vi "Swabian_UI.vi"() -> ()   [LabVIEW 2018]
uses:
  swabian_vis/swabian_channel_settings.ctl
  swabian_vis/channel_settings.ctl
  swabian_vis/reference_checkbox_tdef.ctl
  swabian_vis/stream_modes.ctl
  swabian_vis/swabian_q_tdef.ctl
  swabian_vis/swabian_actions.ctl
  swabian_vis/swabian_local_data_tdef.ctl
  swabian_vis/swabian_events_tdef.ctl
  swabian_vis/update_chart_tdef.ctl
  swabian_vis/channel_data_tdef.ctl
  swabian_vis/swabian_buffer_tdef.ctl
  swabian_vis/leftovers_struct.ctl
  swabian_vis/swabian_hisotgram_settings.ctl
  C:/Users/SWIR TCSPC/Desktop/Swabian/lib/TTCSharp32.dll
  lib/TTCSharp32.dll
panel:
  out "status":string="Status: " caption="Status"
  in  "connect":bool
  in  "experiments":T1(tab)
  in  "Trigger edge":bool[](array[boolean])=[FALSE, FALSE, FALSE, FALSE, FALSE, FALSE, FALSE, FALSE]
  in  "Channels to chart":bool[](array[boolean])=[FALSE, FALSE, FALSE, FALSE, FALSE, FALSE, FALSE, FALSE]
  in  "save_settings":bool
  in  "swabian_channel_settings":T2=[{"Threshold (V)"=0.5, "Input Delay (ps)"=0, "Dead Time (ps)"=6000}, {"Threshold (V)"=0.5, "Input Delay (ps)"=0, "Dead Time (ps)"=6000}, {"Threshold (V)"=0.5, "Input Delay (ps)"=0, "Dead Time (ps)"=6000}, {"Threshold (V)"=0.5, "Input Delay (ps)"=0, "Dead Time (ps)"=6000}, {"Threshold (V)"=0.5, "Input Delay (ps)"=0, "Dead Time (ps)"=6000}, {"Threshold (V)"=0.5, "Input Delay (ps)"=0, "Dead Time (ps)"=6000}, {"Threshold (V)"=0.5, "Input Delay (ps)"=0, "Dead Time (ps)"=6000}, {"Threshold (V)"=0.5, "Input Delay (ps)"=0, "Dead Time (ps)"=6000}] {"Dead Time (ps)" min=0 step=6000; "Threshold (V)" min=0.0 max=2.5 step=0.1}
  in  "chart_counts":bool
  in  "Trigger \nedge":bool[](array[boolean])=[FALSE, FALSE, FALSE, FALSE, FALSE, FALSE, FALSE, FALSE]
  in  "check_sync":bool
  in  "Time (sec)":i64=10 min=1
  in  "Stream Mode":T4
  in  "Notes":string caption="Status"
  in  "Data Path":path=path "C:/Users/SWIR TCSPC/Desktop/Swabian/test_data/test1.photons"
  in  "Channels\nto Stream":bool[](array[boolean])=[TRUE, TRUE, FALSE, FALSE, FALSE, FALSE, FALSE, FALSE]
  in  "stream_to_file":bool
  in  "Reference\nChannel":T5=enum."ch0"
  in  "Sync Rate (Hz)":dbl=40000000.0 min=0.0
  in  "n_bins":i32=100 caption="Number of Bins" min=0
  in  "stop_time":dbl=100.0 caption="Stop time (ns)" min=0.001 max=1000000000.0
  in  "start_time":dbl=1.0 caption="Start Time (ns)" min=0.001 max=1000000000.0
  in  "Time (sec)":i64=1 min=1
  in  "Stream Mode":T4
  in  "Notes":string="Status: " caption="Status"
  in  "Data Path":path=path "C:/Users/bspoka/Desktop/phot_test.photons"
  in  "Channels to\nHistogram":bool[](array[boolean])=[FALSE, FALSE, FALSE, FALSE, FALSE, FALSE, FALSE, FALSE]
  in  "plot_lifetimes":bool
  in  "Reference\nChannel":T5
  in  "sync_rate_histo":i32 caption="Sync Rate (Hz)" min=0
  in  "plots":enum32{"chart", "xy_graph"}(tab)
  out "counts_chart":T6(graph)
  out "Counts/sec":T6
  in  "save_chart_data":bool
  out "xy_graph":cluster{dbl[], dbl[]}[](graph)
  # "0"
  # "1"
  # "2"
  # "3"
  # "4"
  # "5"
  # "6"
  # "7"
  # "Threshold (V)"
  # "Delay (ps)"
  # "Dead Time (ps)"
  # "Ch 0"
  # "Ch 1"
  # "Ch 2"
  # "Ch 3"
  # "Ch 4"
  # "Ch 5"
  # "Ch 6"
  # "Ch 7"
  # "0"
  # "1"
  # "2"
  # "3"
  # "4"
  # "5"
  # "6"
  # "7"
  # "0"
  # "1"
  # "2"
  # "3"
  # "4"
  # "5"
  # "6"
  # "7"
  # "0"
  # "1"
  # "2"
  # "3"
  # "4"
  # "5"
  # "6"
  # "7"
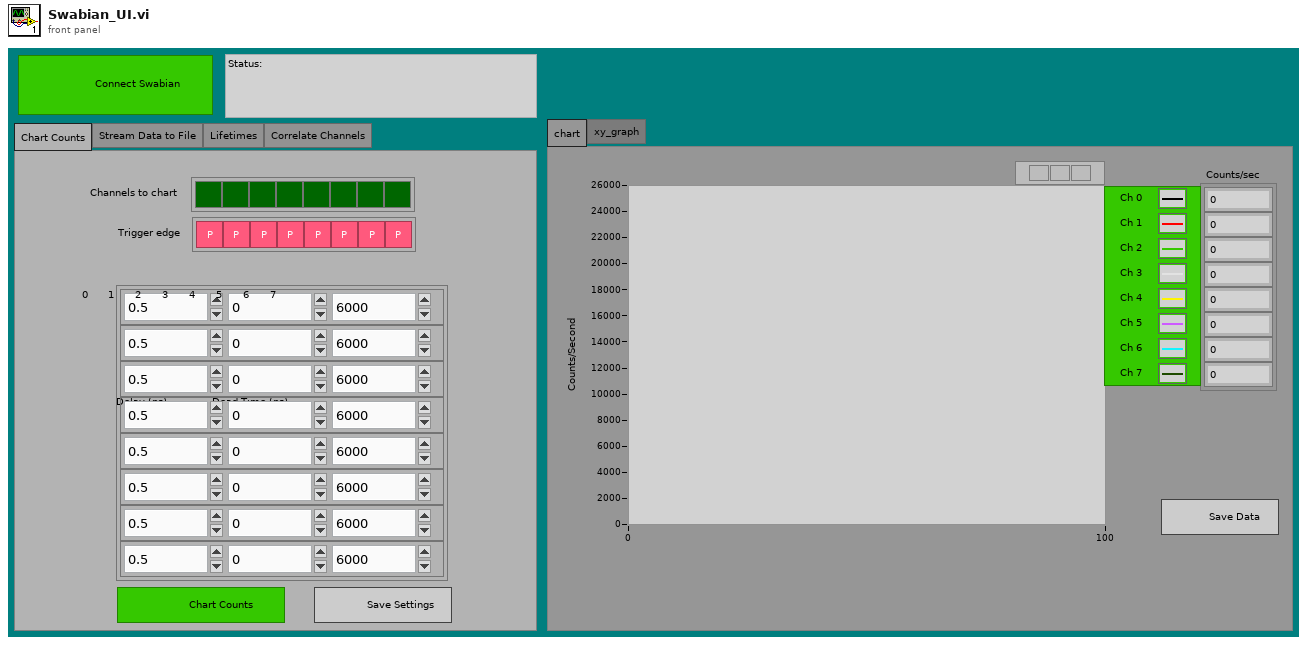
[diagram p1: front panel]
types:
  T1 = enum32{"Chart Counts", "Stream Data to File", "Lifetimes", "Correlate Channels"}
  T2 = typedef "swabian_channel_settings.ctl" = T3[]
  T3 = typedef "channel_settings.ctl" = cluster{"Threshold (V)":dbl, "Input Delay (ps)":i64, "Dead Time (ps)":i64}
  T4 = typedef "stream_modes.ctl" = enum16{"Time (s)"}
  T5 = typedef "reference_checkbox_tdef.ctl" = enum32{"No Selection", "ch0", "ch1", "ch2", "ch3", "ch4", "ch5", "ch6", "ch7"}
  T6 = cluster{"counts_chart":dbl, "counts_chart 2":dbl, "counts_chart 3":dbl, "counts_chart 4":dbl, "counts_chart 5":dbl, "counts_chart 6":dbl, "counts_chart 7":dbl, "counts_chart 8":dbl}
  T7 = typedef "swabian_local_data_tdef.ctl" = cluster{"events":T8, "stop_q":refnum<queue>, "tagger_reference":refnum<k24>, "connect_button":refnum<vi>, "counter_reference":refnum<k24>, "tagger_stream_reference":refnum<k24>, "log_reference":refnum<file>, "current_log_offset":i64, "tt20_buffer_q":refnum<queue>, "stream_to_file_button":refnum<vi>, "num_records":u64, "connected?":bool, "plots":refnum<vi>, "histogram_bin_edges":i64[], "histogrammer":refnum<k24>, "plot_lifetimes":refnum<vi>, "xy_graph":refnum<vi>, "Reference\nChannel":T5, "trigger_channels":i32[], "filter_channels":i32[], "active_channels":i32[], "acq_mode":i32, "Reference\nChannel":T5, "acq_time":i64, "leftovers":T9, "sync_period_ps":i64, "raw_stream_path":path, "Leftovers":cluster{"missing_sync_data":u64[], "missing_events":i32}, "first_batch":i32, "first_sync_stamp":u64}
  T8 = typedef "swabian_events_tdef.ctl" = cluster{"update_status":refnum<user-event>, "update_chart":refnum<user-event>, "update_xy":refnum<user-event>, "send_channel_data":refnum<user-event>}
  T9 = typedef "leftovers_struct.ctl" = cluster{"leftover_stamps":i64[], "leftover_channels":i32[], "any?":bool}
  T10 = typedef "swabian_q_tdef.ctl" = cluster{"action":T11, "data":variant}
  T11 = typedef "swabian_actions.ctl" = enum16{"connect", "disconnect", "chart_counts", "stop_chart", "stream_to_file", "correlate_channels", "plot_histogram", "exit_prog", "apply_channel_settings", "save_chart_data", "save_graph_data", "check_sync", "disco_party"}
  T12 = typedef "swabian_event_refs.ctl" = cluster{"event registration refnum":refnum<event-registration>, "Event Registration Refnum 2":refnum<event-registration>, "Event Registration Refnum 3":refnum<event-registration>, "Event Registration Refnum 4":refnum<event-registration>}
  T13 = typedef "swabian_hisotgram_settings.ctl" = cluster{"start_time(10^s)":dbl, "stop_time(10^s)":dbl, "start_channel":T5, "stop-channel":T5, "n_bins":i32, "Channels to\nHistogram":bool[]}
  T14 = cluster{"counts_chart":dbl, "counts_chart 2":dbl, "counts_chart 3":dbl, "counts_chart 4":dbl, "counts_chart 5":dbl, "counts_chart 6":dbl, "counts_chart 7":dbl, "counts_chart 8":dbl}[]
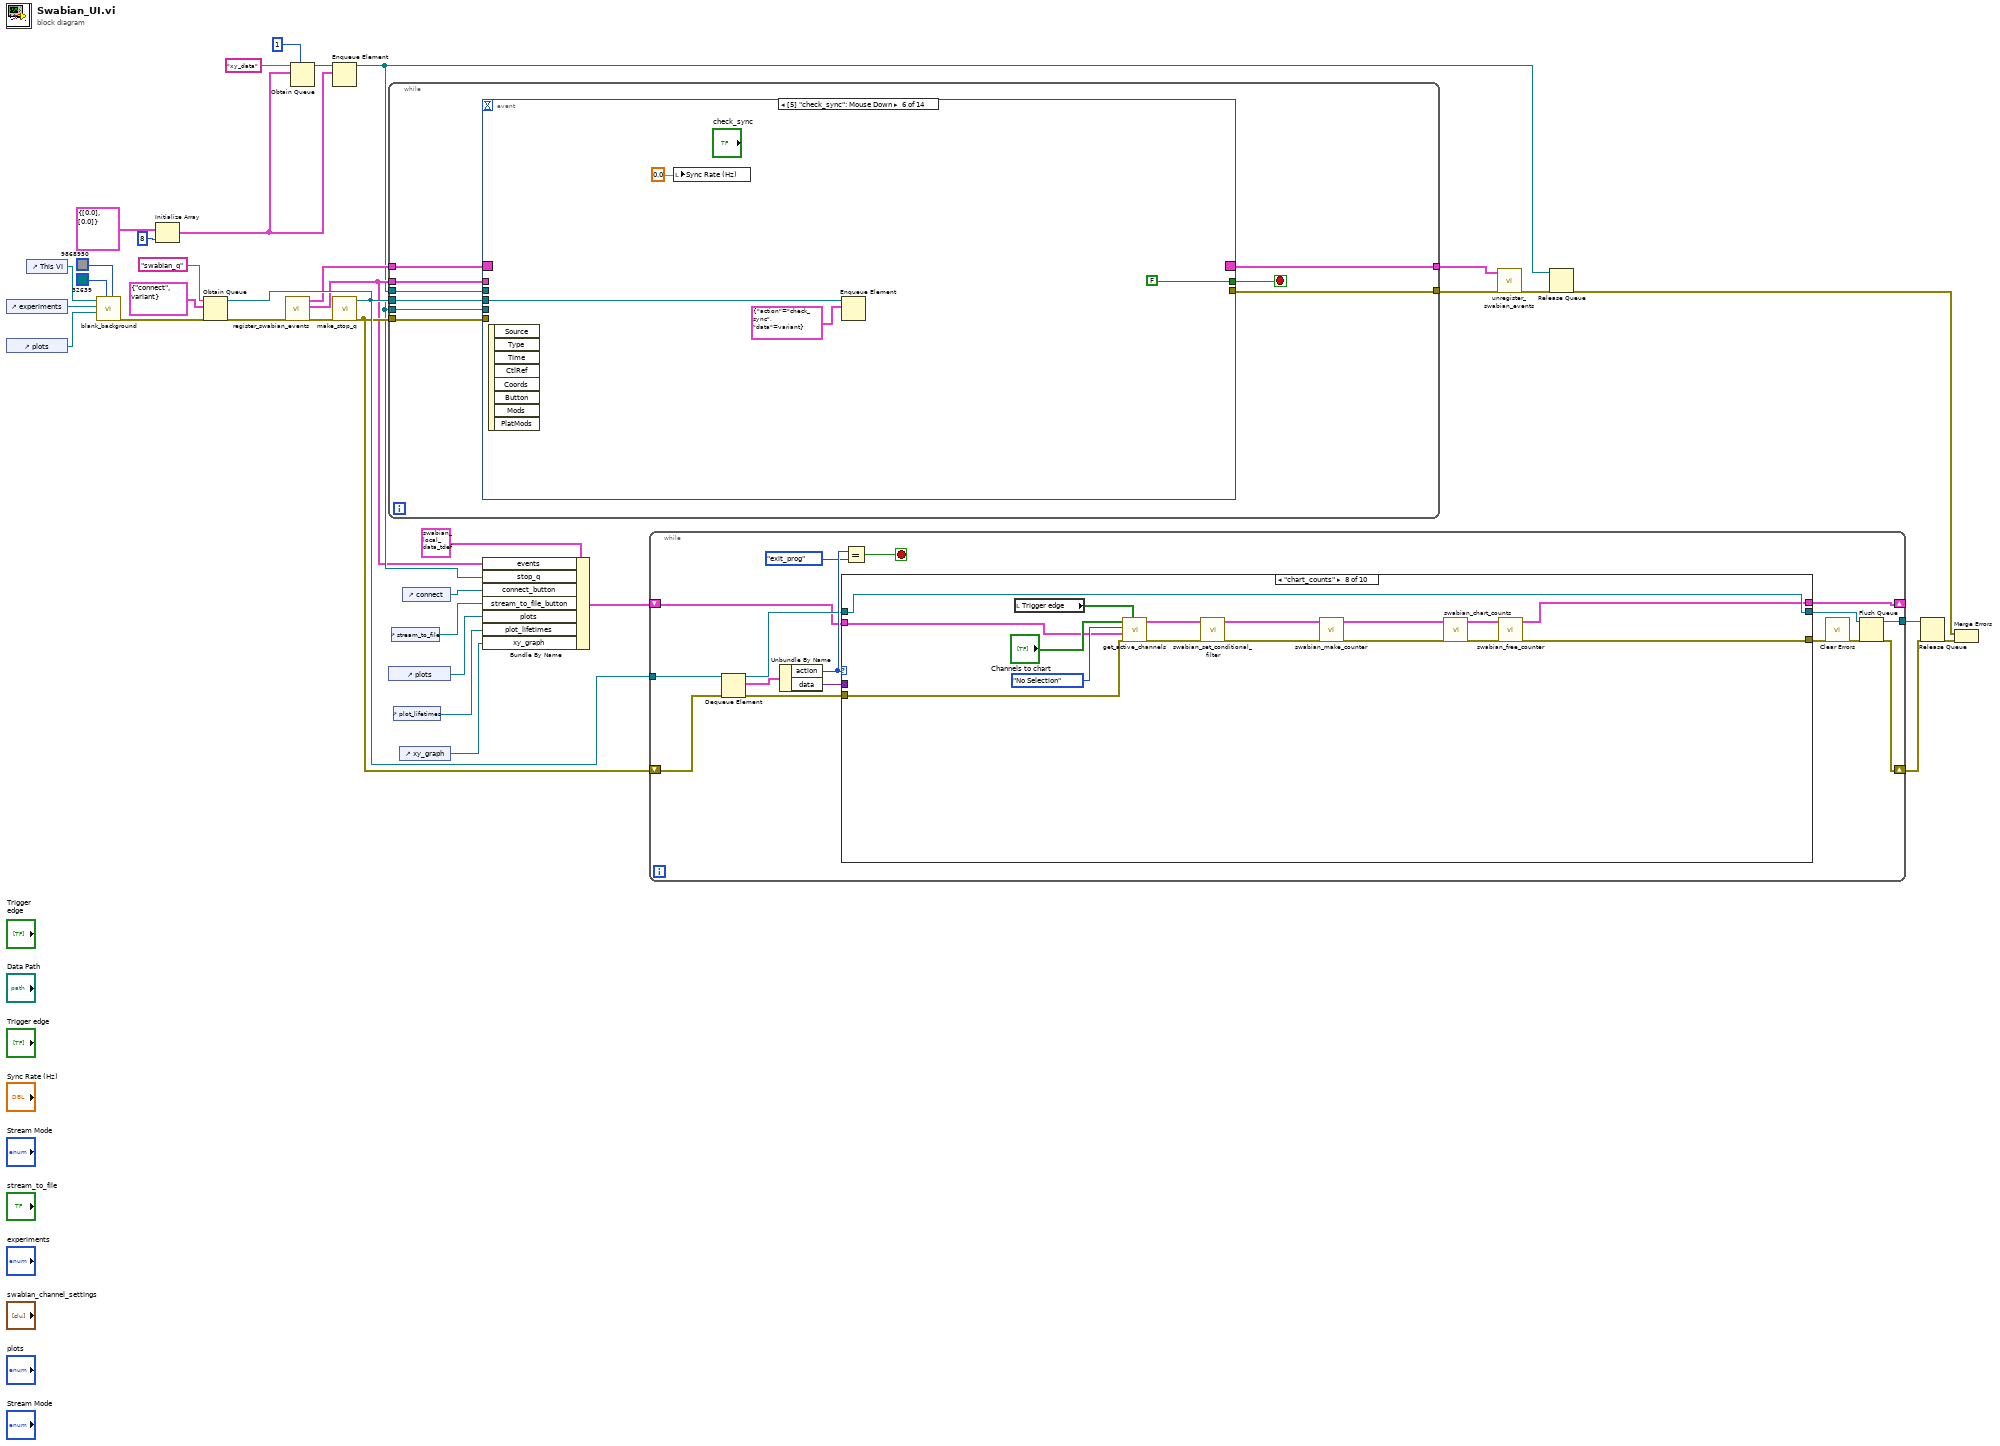
[diagram p0: block diagram]
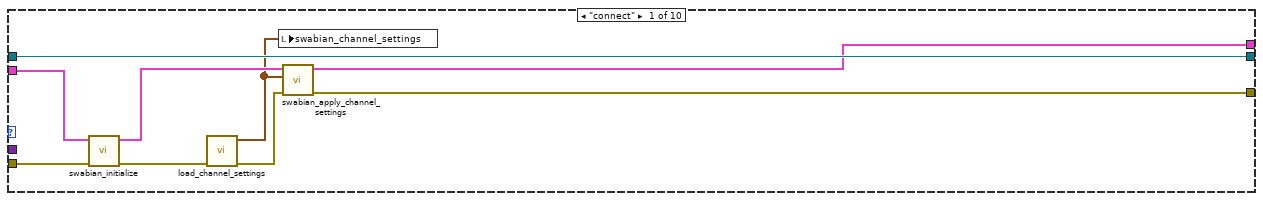
[diagram p2: hidden frame]
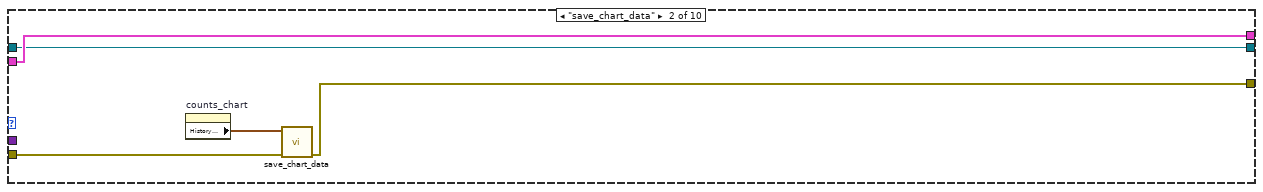
[diagram p3: hidden frame]
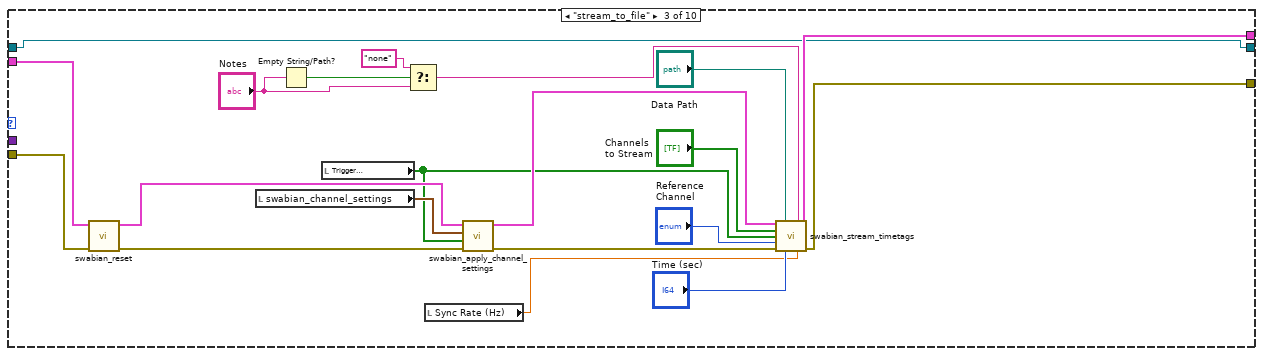
[diagram p4: hidden frame]
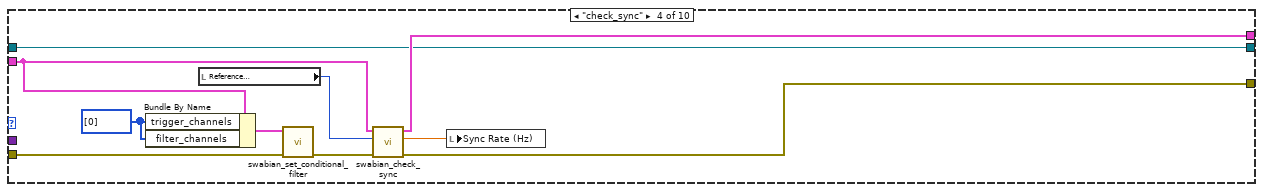
[diagram p5: hidden frame]
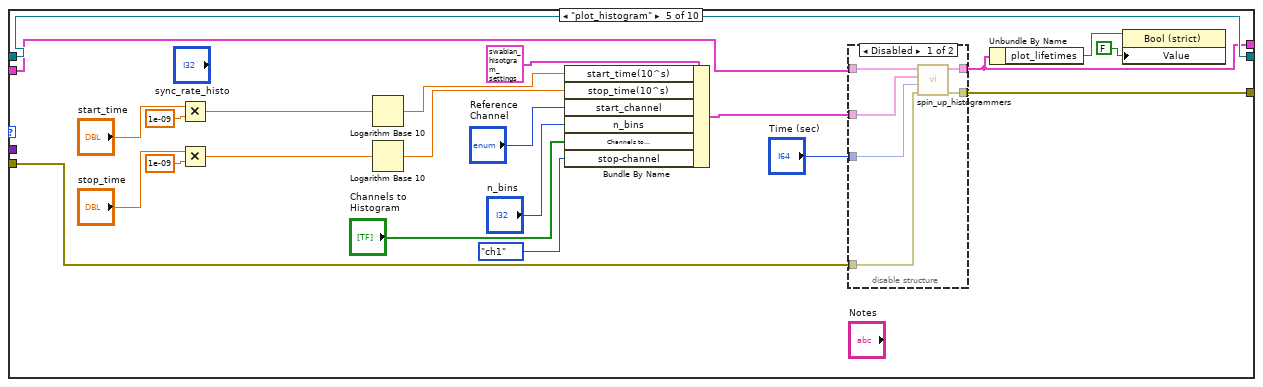
[diagram p6: hidden frame]
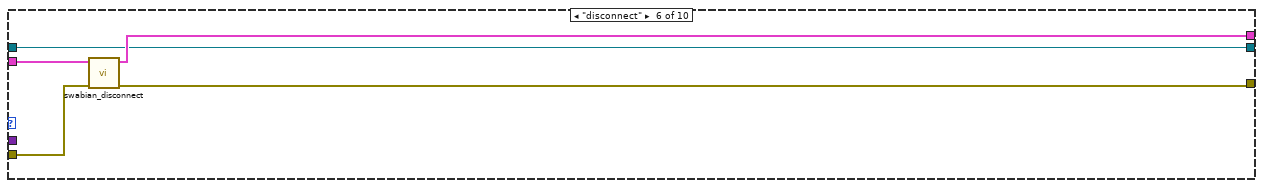
[diagram p8: hidden frame]
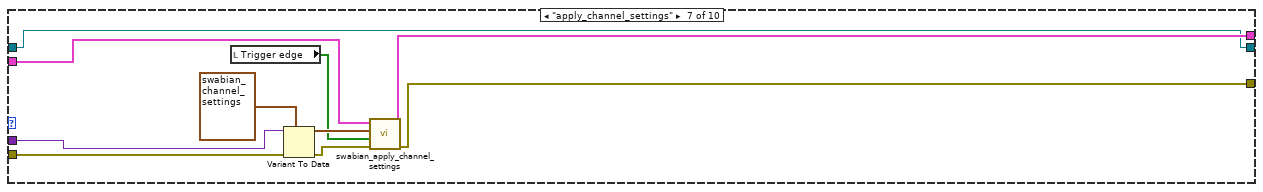
[diagram p9: hidden frame]
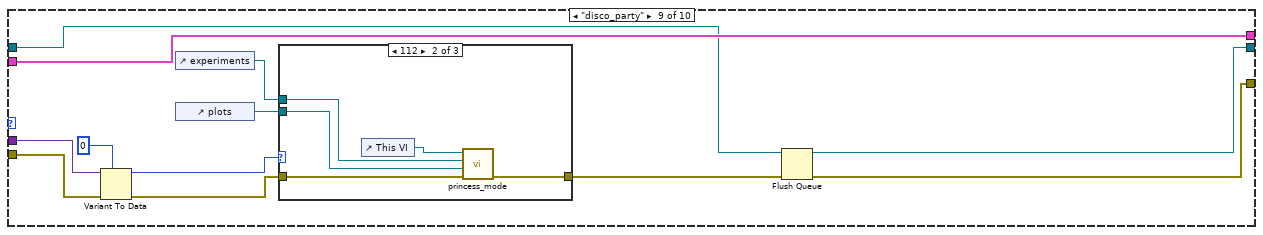
[diagram p10: hidden frame]
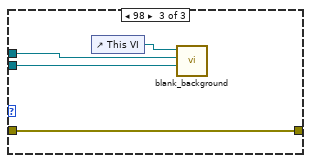
[diagram p12: hidden frame]
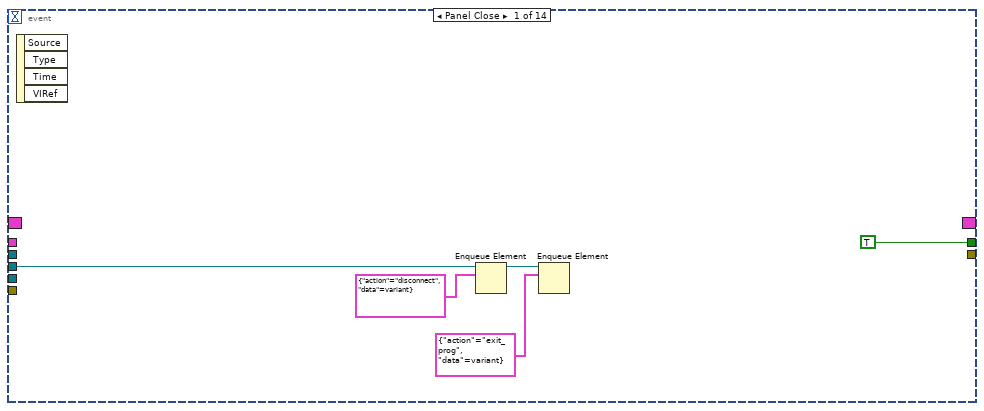
[diagram p14: hidden frame]
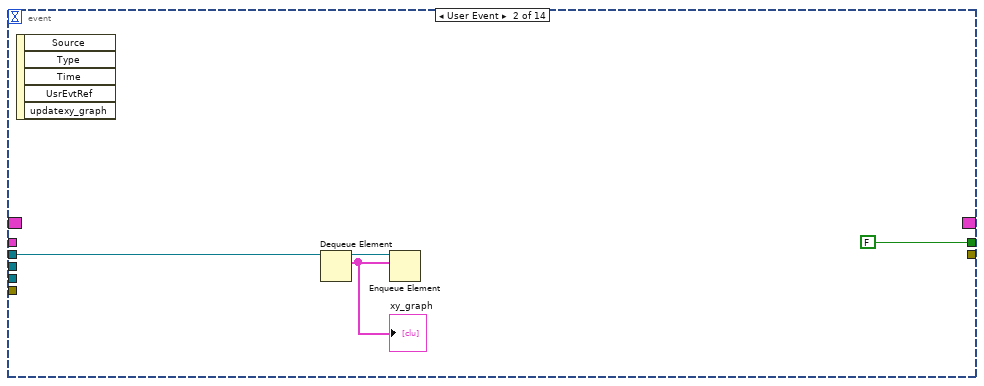
[diagram p15: hidden frame]
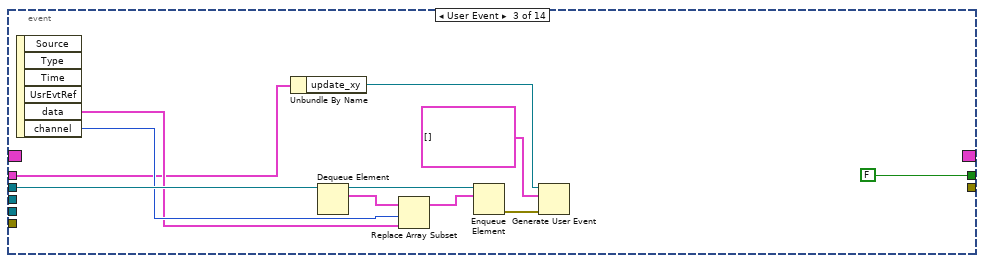
[diagram p16: hidden frame]
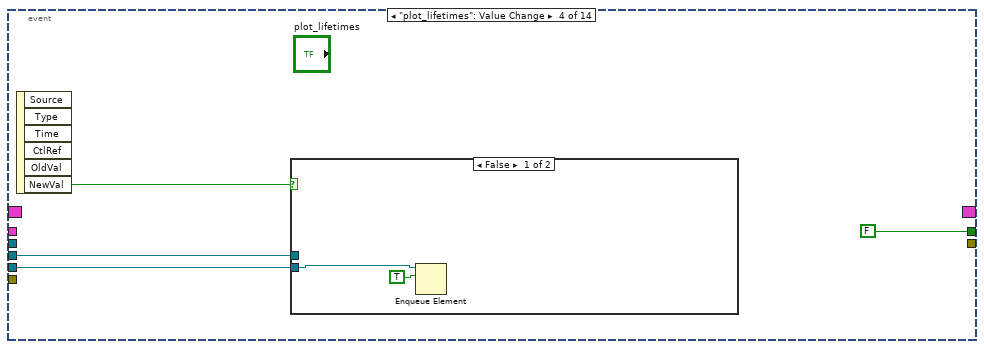
[diagram p17: hidden frame]
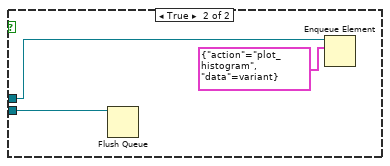
[diagram p18: hidden frame]
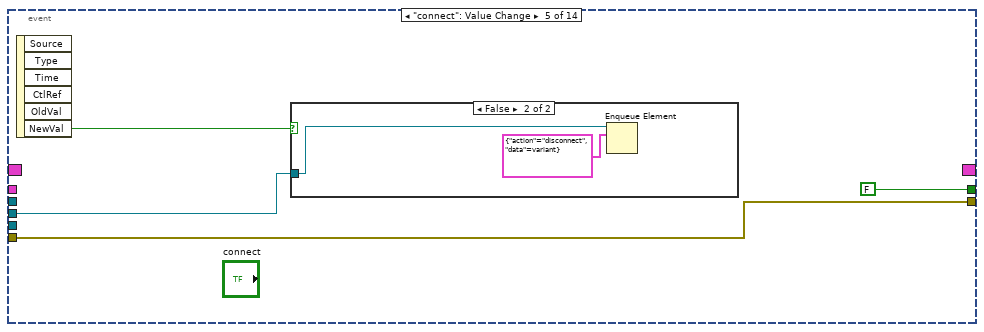
[diagram p19: hidden frame]
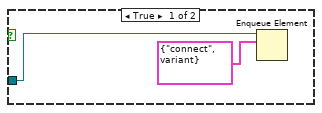
[diagram p20: hidden frame]
diagram:
  n1 = control-ref of="experiments"() -> (w13:refnum<vi>)
  n2 = control-ref of="plots"() -> (w17:refnum<vi>)
  n3 = control-ref of="This VI"() -> (w18:refnum<vi>)
  n4 = call "blank_background.vi"(5:"plots"=u32 9868950 ("plots"), "backg"=u32 32639, 9:"plots"=w17, "experiments 2"=w13, "VI in"=w18) -> ("error in (no error) 2"=w19:errorcluster)  [unwired: 6 in]
  n5 = Initialize Array(cluster{dbl[], dbl[]} {[0.0], [0.0]}, 8 ("dimension size")) -> (w1:cluster{dbl[], dbl[]}[])
  n6 = Obtain Queue(name (unnamed)="swabian_q", element data type=T10 {"action"=enum."connect", "data"=variant} ("output cluster"), error in (no error)=w19) -> (queue out=w34:refnum<queue>, error out=w31:errorcluster)  [unwired: 2 in, 1 out]
  n7 = call "register_swabian_events.vi"("error in (no error)"=w31) -> ("error out"=w24:errorcluster, "events"=w4:T8, "references"=w28:T12)  [unwired: 8 in]
  n8 = Obtain Queue(max queue size (-1, unlimited)=1, name (unnamed)="xy_data", element data type=w1) -> (queue out=w3:refnum<queue>)  [unwired: 2 in, 2 out]
  n9 = Enqueue Element(queue=w3, element=w1) -> (queue out=w2:refnum<queue>)  [unwired: 2 in, 2 out]
  n10 = call "make_stop_q.vi"("error in (no error)"=w24) -> ("error out"=w23:errorcluster, "stop_q"=w22:refnum<queue>)  [unwired: 9 in]
  n11 = while {
    tunnel: w34 -> [w45]
    tunnel: w28 -> [w37]
    tunnel: w23 -> [w43]
    tunnel: [w42] -> w27
    tunnel: [w41] -> w26
    tunnel: w22 -> [w40]
    tunnel: w2 -> [w39]
    tunnel: w4 -> [w38]
    stop <- w44 stop-if-true
    n12 = event shown="[5] \"check_sync\": Mouse Down" {
      selector: w37 -> [_ _ _ _ _ _ _ _ _ _ _ _ _ _]
      dyn-events: [_ _ _ _ _ _ _ _ _ _ _ _ _ _] -> w41
      timeout: _ -> [_ _ _ _ _ _ _ _ _ _ _ _ _ _]
      tunnel: w45 -> [w50 _ _ w67 w77 w85 _ w92 _ w114 w118 w129 w137 _]
      tunnel: [TRUE FALSE FALSE FALSE FALSE FALSE FALSE _ FALSE FALSE FALSE FALSE FALSE FALSE] -> w44
      tunnel: w43 -> [_ _ _ _ w75 _ w89 _ w100 w112 w116 w130 w133 w139]
      tunnel: [_ _ _ _ w75 _ w88 _ w100 w112 w116 w130 w133 w139] -> w42
      tunnel: w40 -> [_ _ _ w68 _ _ _ w91 _ _ w117 _ _ _]
      tunnel: w39 -> [_ w53 w64 _ _ _ _ _ _ _ _ _ _ _]
      tunnel: w38 -> [_ _ w56 _ _ _ _ _ _ _ _ _ _ _]
      event Panel Close {
        n13 = event-data() -> ()  [unwired: 1 in, 4 out]
        n14 = Enqueue Element(queue=w50, element=T10 {"action"=enum."disconnect", "data"=variant}) -> (queue out=w47:refnum<queue>)  [unwired: 2 in, 2 out]
        n15 = Enqueue Element(queue=w47, element=T10 {"action"=enum."exit_prog", "data"=variant}) -> ()  [unwired: 2 in, 3 out]
      }
      event User Event {
        n16 = event-data() -> ()  [unwired: 1 in, 5 out]
        n17 = Dequeue Element(queue=w53) -> (queue out=w52:refnum<queue>, element=w51:cluster{dbl[], dbl[]}[])  [unwired: 2 in, 2 out]
        "xy_graph" <- w51
        n18 = Enqueue Element(queue=w52, element=w51) -> ()  [unwired: 2 in, 3 out]
      }
      event User Event {
        n19 = event-data() -> ("data"=w61:cluster{dbl[], dbl[]}, "channel"=w62:u8)  [unwired: 1 in, 4 out]
        n20 = Unbundle By Name(w56) -> ("update_xy"=w55:refnum<user-event>)
        n21 = Dequeue Element(queue=w64) -> (queue out=w60:refnum<queue>, element=w63:cluster{dbl[], dbl[]}[])  [unwired: 2 in, 2 out]
        n22 = Replace Array Subset(array=w63, new element=w61, index=w62) -> (w59:cluster{dbl[], dbl[]}[])
        n23 = Enqueue Element(queue=w60, element=w59) -> (error out=w57:errorcluster)  [unwired: 2 in, 2 out]
        n24 = Generate User Event(user event=w55, event data cluster=cluster{dbl[], dbl[]}[] [] ("event data"), error in=w57) -> ()  [unwired: 1 in, 2 out]
      }
      event "plot_lifetimes": Value Change {
        n25 = event-data() -> ("NewVal"=w69:bool)  [unwired: 1 in, 5 out]
        n26 = case shown="False" w69 {
          tunnel: w68 -> [w71 w74]
          tunnel: w67 -> [_ w73]
          frame False {
            n27 = Enqueue Element(queue=w71, element=TRUE) -> ()  [unwired: 2 in, 3 out]
          }
          frame True {
            n28 = Flush Queue(queue=w74) -> ()  [unwired: 1 in, 3 out]
            n29 = Enqueue Element(queue=w73, element=T10 {"action"=enum."plot_histogram", "data"=variant}) -> ()  [unwired: 2 in, 3 out]
          }
        }
      }
      event "connect": Value Change {
        n30 = event-data() -> ("NewVal"=w78:bool)  [unwired: 1 in, 5 out]
        n31 = case shown="False" w78 {
          tunnel: w77 -> [w80 w82]
          frame True {
            n32 = Enqueue Element(queue=w80, element=T10 {"action"=enum."connect", "data"=variant}) -> ()  [unwired: 2 in, 3 out]
          }
          frame False {
            n33 = Enqueue Element(queue=w82, element=T10 {"action"=enum."disconnect", "data"=variant}) -> ()  [unwired: 2 in, 3 out]
          }
        }
      }
      event "check_sync": Mouse Down {
        n34 = event-data() -> ()  [unwired: 1 in, 8 out]
        n35 = local write "Sync Rate (Hz)"(0.0 ("Sync Rate (Hz)")) -> ()
        n36 = Enqueue Element(queue=w85, element=T10 {"action"=enum."check_sync", "data"=variant}) -> ()  [unwired: 2 in, 3 out]
      }
      event "save_settings": Mouse Down {
        n37 = event-data() -> ()  [unwired: 1 in, 6 out]
        n38 = local read "swabian_channel_settings"() -> (w90:T2)
        n39 = call "save_channel_settings.vi"("error in"=w89, "swabian_channel_settings"=w90) -> ("error out"=w88:errorcluster)  [unwired: 9 in]
      }
      event "chart_counts": Value Change {
        n40 = event-data() -> ("NewVal"=w93:bool)  [unwired: 1 in, 5 out]
        n41 = case shown="True" w93 {
          tunnel: w92 -> [_ w98]
          tunnel: w91 -> [w95 w96]
          frame False {
            n42 = Enqueue Element(queue=w95, element=TRUE) -> ()  [unwired: 2 in, 3 out]
          }
          frame True {
            n43 = Flush Queue(queue=w96) -> ()  [unwired: 1 in, 3 out]
            n44 = Enqueue Element(queue=w98, element=T10 {"action"=enum."chart_counts", "data"=variant}) -> ()  [unwired: 2 in, 3 out]
          }
        }
      }
      event User Event {
        n45 = event-data() -> ("ch0"=w109:dbl, "ch1"=w108:dbl, "ch2"=w107:dbl, "ch3"=w106:dbl, "ch4"=w105:dbl, "ch5"=w104:dbl, "ch6"=w103:dbl, "ch7"=w102:dbl)  [unwired: 1 in, 4 out]
        n46 = Bundle(cluster=T6 {"counts_chart"=0.0, "counts_chart 2"=0.0, "counts_chart 3"=0.0, "counts_chart 4"=0.0, "counts_chart 5"=0.0, "counts_chart 6"=0.0, "counts_chart 7"=0.0, "counts_chart 8"=0.0} ("counts_chart"), "counts_chart"=w109, "counts_chart 2"=w108, "counts_chart 3"=w107, "counts_chart 4"=w106, "counts_chart 5"=w105, "counts_chart 6"=w104, "counts_chart 7"=w103, "counts_chart 8"=w102) -> (→"counts_chart" →"Counts/sec":T6)
      }
      event "save_chart_data": Mouse Down {
        n47 = event-data() -> ()  [unwired: 1 in, 8 out]
        n48 = Enqueue Element(queue=w114, element=T10 {"action"=enum."save_chart_data", "data"=variant}) -> ()  [unwired: 2 in, 3 out]
      }
      event "stream_to_file": Value Change {
        n49 = event-data() -> ("NewVal"=w119:bool)  [unwired: 1 in, 5 out]
        n50 = case shown="False" w119 {
          tunnel: w118 -> [_ w124]
          tunnel: w117 -> [w121 w122]
          frame False {
            n51 = Enqueue Element(queue=w121, element=TRUE) -> ()  [unwired: 2 in, 3 out]
          }
          frame True {
            n52 = Flush Queue(queue=w122) -> ()  [unwired: 1 in, 3 out]
            n53 = Enqueue Element(queue=w124, element=T10 {"action"=enum."stream_to_file", "data"=variant}) -> ()  [unwired: 2 in, 3 out]
          }
        }
      }
      event event type 5.0.x8000000b {
        n54 = event-data() -> ("Char"=w127:i16)  [unwired: 1 in, 9 out]
        n55 = Bundle By Name(cluster=T10 {"action"=enum."disco_party", "data"=variant} ("element"), "data"=w127) -> (w126:T10)
        n56 = Enqueue Element(queue=w129, element=w126) -> ()  [unwired: 2 in, 3 out]
        n57 = event-data("Discard?"=TRUE) -> ()  [unwired: 2 in, 1 out]
      }
      event Value Change {
        n58 = event-data() -> ("NewVal"=w134:T2)  [unwired: 1 in, 5 out]
        n59 = Bundle By Name(cluster=T10 {"action"=enum."apply_channel_settings", "data"=variant} ("element"), "data"=w134) -> (w135:T10)
        n60 = Enqueue Element(queue=w137, element=w135) -> ()  [unwired: 2 in, 3 out]
      }
      event User Event {
        n61 = event-data() -> ("update_status"=→"status":string)  [unwired: 1 in, 4 out]
      }
    }
  }
  n62 = control-ref of="plots"() -> (w16:refnum<vi>)
  n63 = control-ref of="stream_to_file"() -> (w20:refnum<vi>)
  n64 = control-ref of="plot_lifetimes"() -> (w12:refnum<vi>)
  n65 = control-ref of="xy_graph"() -> (w11:refnum<vi>)
  n66 = control-ref of="connect"() -> (w21:refnum<vi>)
  n67 = Bundle By Name(cluster=T7 {"events"={"update_status"=refnum, "update_chart"=refnum, "update_xy"=refnum, "send_channel_data"=refnum}, "stop_q"=refnum, "tagger_reference"=refnum, "connect_button"=refnum, "counter_reference"=refnum, "tagger_stream_reference"=refnum, "log_reference"=refnum, "current_log_offset"=0, "tt20_buffer_q"=refnum, "stream_to_file_button"=refnum, "num_records"=0, "connected?"=FALSE, "plots"=refnum, "histogram_bin_edges"=[], "histogrammer"=refnum, "plot_lifetimes"=refnum, "xy_graph"=refnum, "Reference\nChannel"=enum."ch0", "trigger_channels"=[], "filter_channels"=[], "active_channels"=[], "acq_mode"=0, "Reference\nChannel"=enum."ch0", "acq_time"=0, "leftovers"={"leftover_stamps"=[], "leftover_channels"=[], "any?"=FALSE}, "sync_period_ps"=0, "raw_stream_path"=path "", "Leftovers"={"missing_sync_data"=[], "missing_events"=0}, "first_batch"=0, "first_sync_stamp"=0} ("swabian_local_data"), "events"=w4, "stop_q"=w22, "connect_button"=w21, "stream_to_file_button"=w20, "plots"=w16, "plot_lifetimes"=w12, "xy_graph"=w11) -> (w29:T7)
  n68 = while {
    tunnel: w34 -> [w156]
    shift-right: [w143] -> w32
    shift-left: w23 -> [w154]
    tunnel: [w141] -> w33
    shift-right: [w147] -> _
    shift-left: w29 -> [w148]
    stop <- w150 stop-if-true
    n69 = Dequeue Element(queue=w156, error in (no error)=w154) -> (queue out=w149:refnum<queue>, element=w155:T10, error out=w153:errorcluster)  [unwired: 1 in, 1 out]
    n70 = Unbundle By Name(w155) -> ("action"=w152:T11, "data"=w145:variant)
    n71 = case shown="\"chart_counts\"" w152 {
      tunnel: w153 -> [w165 w169 w180 w195 w207 w233 w242 w252 w271 w284]
      tunnel: [w160 w168 w186 w200 w206 w232 w236 w257 w264 w284] -> w146
      tunnel: w149 -> [w164 w166 w185 w198 w219 w229 w237 w259 w263 w283]
      tunnel: [w164 w166 w185 w198 w219 w229 w237 w259 w262 w283] -> w142
      tunnel: w148 -> [w163 w167 w178 w194 w205 w230 w239 w249 w266 w282]
      tunnel: [w158 w167 w187 w199 w204 w231 w238 w255 w266 w282] -> w147
      tunnel: w145 -> [_ _ _ _ _ _ w243 _ w270 _]
      frame "connect" {
        n72 = call "swabian_initialize.vi"("error in (no error)"=w165, "swabian_local_data_IN"=w163) -> ("error out"=w162:errorcluster, "swabian_local_data"=w159:T7)  [unwired: 8 in]
        n73 = call "load_channel_settings.vi"("error in"=w162) -> ("error out"=w161:errorcluster, "swabian_channel_settings"=w157:T2)  [unwired: 9 in]
        n74 = local write "swabian_channel_settings"(w157) -> ()
        n75 = call "swabian_apply_channel_settings.vi"("error in (no error)"=w161, "swabian_channel_settings"=w157, "swabian_local_data"=w159) -> ("error IO"=w160:errorcluster, "swabian_local_data 2"=w158:T7)  [unwired: 7 in]
      }
      frame "save_chart_data" {
        n76 = property on="counts_chart" class="WFChart (strict)"() -> ("History Data"=w170:T14)  [unwired: 2 in, 2 out]
        n77 = call "save_chart_data.vi"("error in (no error)"=w169, "History Data"=w170) -> ("error out"=w168:errorcluster)  [unwired: 9 in]
      }
      frame "stream_to_file" {
        n78 = call "swabian_reset.vi"("error in (no error)"=w180, "swabian_local_data"=w178) -> ("error IO"=w179:errorcluster, "swabian_local_data 2"=w177:T7)  [unwired: 8 in]
        n79 = local read "swabian_channel_settings"() -> (w181:T2)
        n80 = Empty String/Path?(string/path="Notes") -> (empty?=w174:bool)
        n81 = local read "Trigger \nedge"() -> (w175:bool[])
        n82 = Select(t="none", s=w174, f="Notes") -> (s? t:f=w171:string)
        n83 = local read "Sync Rate (Hz)"() -> (w176:dbl)
        n84 = call "swabian_apply_channel_settings.vi"("error in (no error)"=w179, "Trigger edge"=w175, "swabian_channel_settings"=w181, "swabian_local_data"=w177) -> ("error IO"=w183:errorcluster, "swabian_local_data 2"=w182:T7)  [unwired: 6 in]
        n85 = call "swabian_stream_timetags.vi"("swabian_local_data"=w182, "Data_path"="Data Path", "Notes"=w171, "channels_to_stream"="Channels\nto Stream", "Trigger edge"=w175, "Reference\nChannel"="Reference\nChannel", "error in (no error)"=w183, "acq_time"="Time (sec)", "sync_rate"=w176) -> ("swabian_local_data 2"=w187:T7, "error out"=w186:errorcluster)  [unwired: 5 in]
      }
      frame "check_sync" {
        w193 = i32[] [0] ("trigger_channels")
        n86 = Bundle By Name(cluster=w194, "trigger_channels"=w193, "filter_channels"=w193) -> (w192:T7)
        n87 = local read "Reference\nChannel"() -> (w197:T5)
        n88 = call "swabian_set_conditional_filter.vi"("error in (no error)"=w195, "swabian_local_data_IN"=w192) -> ("error out"=w191:errorcluster)  [unwired: 8 in, 1 out]
        n89 = call "swabian_check_sync.vi"("error in (no error)"=w191, "Reference\nChannel"=w197, "swabian_local_data_IN"=w194) -> ("error out"=w200:errorcluster, "sync_rate_hz"=w196:dbl, "swabian_local_data"=w199:T7)  [unwired: 6 in]
        n90 = local write "Sync Rate (Hz)"(w196) -> ()
      }
      frame "plot_histogram" {
        n91 = Multiply(x="start_time", y=1e-09) -> (x*y=w214:dbl)
        n92 = Multiply(x="stop_time", y=1e-09) -> (x*y=w210:dbl)
        n93 = Logarithm Base 10(1:w214) -> (0:w213:dbl)
        n94 = Logarithm Base 10(1:w210) -> (0:w209:dbl)
        n95 = Bundle By Name(cluster=T13 {"start_time(10^s)"=0.0, "stop_time(10^s)"=0.0, "start_channel"=enum."No Selection", "stop-channel"=enum."No Selection", "n_bins"=0, "Channels to\nHistogram"=[FALSE, FALSE, FALSE, FALSE, FALSE, FALSE, FALSE, FALSE]} ("histo-settings"), "start_time(10^s)"=w213, "stop_time(10^s)"=w209, "start_channel"="Reference\nChannel", "n_bins"="n_bins", "Channels to\nHistogram"="Channels to\nHistogram", "stop-channel"=reference_checkbox_tdef."ch1") -> (w203:T13)
        n96 = disable-structure shown="Disabled" {
          disable-tunnel: w207 -> [w228 _]
          disable-tunnel: [w227 _] -> w206
          disable-tunnel: w205 -> [w226 _]
          disable-tunnel: [w225 _] -> w204
          disable-tunnel: w203 -> [w224 _]
          disable-tunnel: "Time (sec)" -> [w223 _]
          frame Disabled {
            n97 = call "spin_up_histogrammers.vi"("error in (no error)"=w228, "acq_time"=w223, "histo-settings"=w224, "swabian_local_data"=w226) -> ("error out"=w227:errorcluster, "swabian_local_data 2"=w225:T7)  [unwired: 6 in]
          }
          frame Enabled {
          }
        }
        n98 = Unbundle By Name(w204) -> ("plot_lifetimes"=w218:refnum<vi>)
        n99 = property class="Bool (strict)"(reference=w218, "Value"=FALSE) -> ()  [unwired: 1 in, 2 out]
      }
      frame "disconnect" {
        n100 = call "swabian_disconnect.vi"("error in (no error)"=w233, "swabian_local_data_IN"=w230) -> ("error out"=w232:errorcluster, "swabian_local_data"=w231:T7)  [unwired: 8 in]
      }
      frame "apply_channel_settings" {
        n101 = local read "Trigger edge"() -> (w234:bool[])
        n102 = Variant To Data(error in=w242, type=T2 [{"Threshold (V)"=0.5, "Input Delay (ps)"=0, "Dead Time (ps)"=6000}, {"Threshold (V)"=0.5, "Input Delay (ps)"=0, "Dead Time (ps)"=6000}, {"Threshold (V)"=0.5, "Input Delay (ps)"=0, "Dead Time (ps)"=6000}, {"Threshold (V)"=0.5, "Input Delay (ps)"=0, "Dead Time (ps)"=6000}, {"Threshold (V)"=0.5, "Input Delay (ps)"=0, "Dead Time (ps)"=6000}, {"Threshold (V)"=0.5, "Input Delay (ps)"=0, "Dead Time (ps)"=6000}, {"Threshold (V)"=0.5, "Input Delay (ps)"=0, "Dead Time (ps)"=6000}, {"Threshold (V)"=0.5, "Input Delay (ps)"=0, "Dead Time (ps)"=6000}] ("NewVal"), Variant=w243) -> (data=w240:T2, error out=w235:errorcluster)
        n103 = call "swabian_apply_channel_settings.vi"("error in (no error)"=w235, "Trigger edge"=w234, "swabian_channel_settings"=w240, "swabian_local_data"=w239) -> ("error IO"=w236:errorcluster, "swabian_local_data 2"=w238:T7)  [unwired: 6 in]
      }
      frame "chart_counts" {
        n104 = local read "Trigger edge"() -> (w244:bool[])
        n105 = call "get_active_channels.vi"("Trigger edge"=w244, "Error In"=w252, "swabian_local_data"=w249, "Reference\nChannel"=reference_checkbox_tdef."No Selection" ("Reference\nChannel"), "channels_to_stream"="Channels to chart") -> ("Error In 2"=w248:errorcluster, "swabian_local_data 2"=w246:T7)  [unwired: 5 in]
        n106 = call "swabian_set_conditional_filter.vi"("error in (no error)"=w248, "swabian_local_data_IN"=w246) -> ("error out"=w247:errorcluster, "swabian_local_data"=w245:T7)  [unwired: 8 in]
        n107 = call "swabian_make_counter.vi"("error in (no error)"=w247, "swabian_local_data_IN"=w245) -> ("error out"=w253:errorcluster, "swabian_local_data"=w254:T7)  [unwired: 8 in]
        n108 = call "swabian_chart_counts.vi"("error in (no error)"=w253, "swabian_local_data"=w254) -> ("error IO"=w258:errorcluster, "swabian_local_data 2"=w256:T7)  [unwired: 8 in]
        n109 = call "swabian_free_counter.vi"("error in (no error)"=w258, "swabian_local_data_IN"=w256) -> ("error out"=w257:errorcluster, "swabian_local_data"=w255:T7)  [unwired: 8 in]
      }
      frame "disco_party" {
        n110 = Variant To Data(error in=w271, type=i16 0 ("Char"), Variant=w270) -> (data=w268:i16, error out=w267:errorcluster)
        n111 = control-ref of="experiments"() -> (w260:refnum<vi>)
        n112 = control-ref of="plots"() -> (w261:refnum<vi>)
        n113 = case shown="112" w268 {
          tunnel: w267 -> [w272 w276 w280]
          tunnel: [w272 w275 w280] -> w265
          tunnel: w261 -> [_ w274 w278]
          tunnel: w260 -> [_ w273 w279]
          frame Default {
          }
          frame 112 {
            n114 = control-ref of="This VI"() -> (w277:refnum<vi>)
            n115 = call "princess_mode.vi"("error out"=w276, "plots"=w274, "experiments 2"=w273, "VI in"=w277) -> ("error out 2"=w275:errorcluster)  [unwired: 7 in]
          }
          frame 98 {
            n116 = control-ref of="This VI"() -> (w281:refnum<vi>)
            n117 = call "blank_background.vi"("plots"=w278, "experiments 2"=w279, "VI in"=w281) -> ()  [unwired: 8 in, 1 out]
          }
        }
        n118 = Flush Queue(queue=w263, error in (no error)=w265) -> (queue out=w262:refnum<queue>, error out=w264:errorcluster)  [unwired: 1 out]
      }
      frame "exit_prog", Default {
      }
    }
    n119 = Equal?(x=w152, y=swabian_actions."exit_prog") -> (x = y?=w150:bool)
    n120 = call <vilib>:"Clear Errors.vi"("error in (no error)"=w146) -> ("error out"=w144:errorcluster)  [unwired: 5 in, 1 out]
    n121 = Flush Queue(queue=w142, error in (no error)=w144) -> (queue out=w141:refnum<queue>, error out=w143:errorcluster)  [unwired: 1 out]
  }
  n122 = call "unregister_swabian_events.vi"("error in (no error)"=w27, "references"=w26) -> ("error out"=w8:errorcluster)  [unwired: 9 in]
  n123 = Release Queue(queue=w2, error in (no error)=w8) -> (error out=w7:errorcluster)  [unwired: 1 in, 2 out]
  n124 = Release Queue(queue=w33, error in (no error)=w32) -> (error out=w25:errorcluster)  [unwired: 1 in, 2 out]
  n125 = Merge Errors(w7, w25) -> ()  [unwired: 1 out]
